vi "PicoCreatePicoMultiBuffers.vi"(1 "Number of Buffers":i32=1, 2 "Buffer and Transfer Settings":T2={"startIndex"=0, "Samples"=1000, "Down Sample Ratio"=1, "Down-Sample Mode"=1} {"Down-Sample Mode" items=["None"=2147483648, "Aggregate"=1, "Decimate"=2, "Average"=4]; "Down Sample Ratio" step=1; "Samples" format="%_6p"}, 3 "enabled array":i16[](array[numeric]), 5 "Data Pointers In":T1, 11 "error in (no error)":errorcluster) -> (6 "Data Pointers":T1, 15 "error out":errorcluster)   [LabVIEW 2024]
doc: "Creates Multiple memory buffers for Pico block and Rapid block examples as configured."
uses:
  PicoBuffers.ctl
panel:
  in  "Dummy enabled array":i16[](array[numeric])=[1, 1, 1, 1, 1, 1, 1, 1, 1, 1]
  # "Samples can be equal to or less\nTotal Pre and Post Trigger Samples"
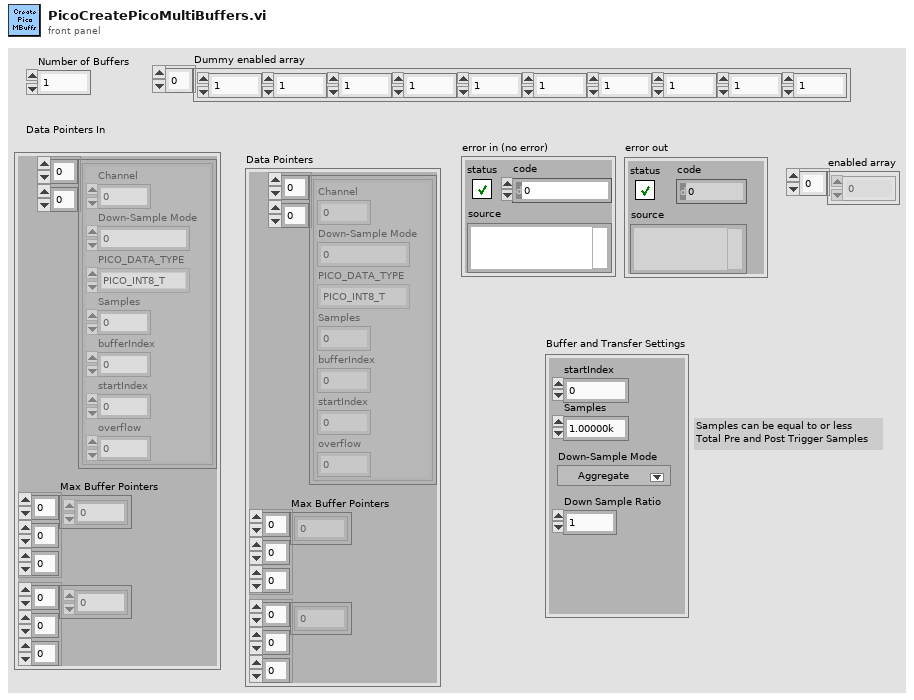
[diagram p1: front panel]
types:
  T1 = typedef "PicoBuffers.ctl" = cluster{"Max Buffer Pointers":u64[][][], "Min Buffer Pointers":u64[][][], "StreamingDataInfo":cluster{"Channel":u32, "Down-Sample Mode":u32, "PICO_DATA_TYPE":enum32{"PICO_INT8_T", "PICO_INT16_T", "PICO_INT32_T", "PICO_UINT32_T", "PICO_INT64_T", ""}, "Samples":i32, "bufferIndex":u64, "startIndex":i32, "overflow":i16}[][]}
  T2 = cluster{"startIndex":u64, "Samples":u64, "Down Sample Ratio":u64, "Down-Sample Mode":u32}
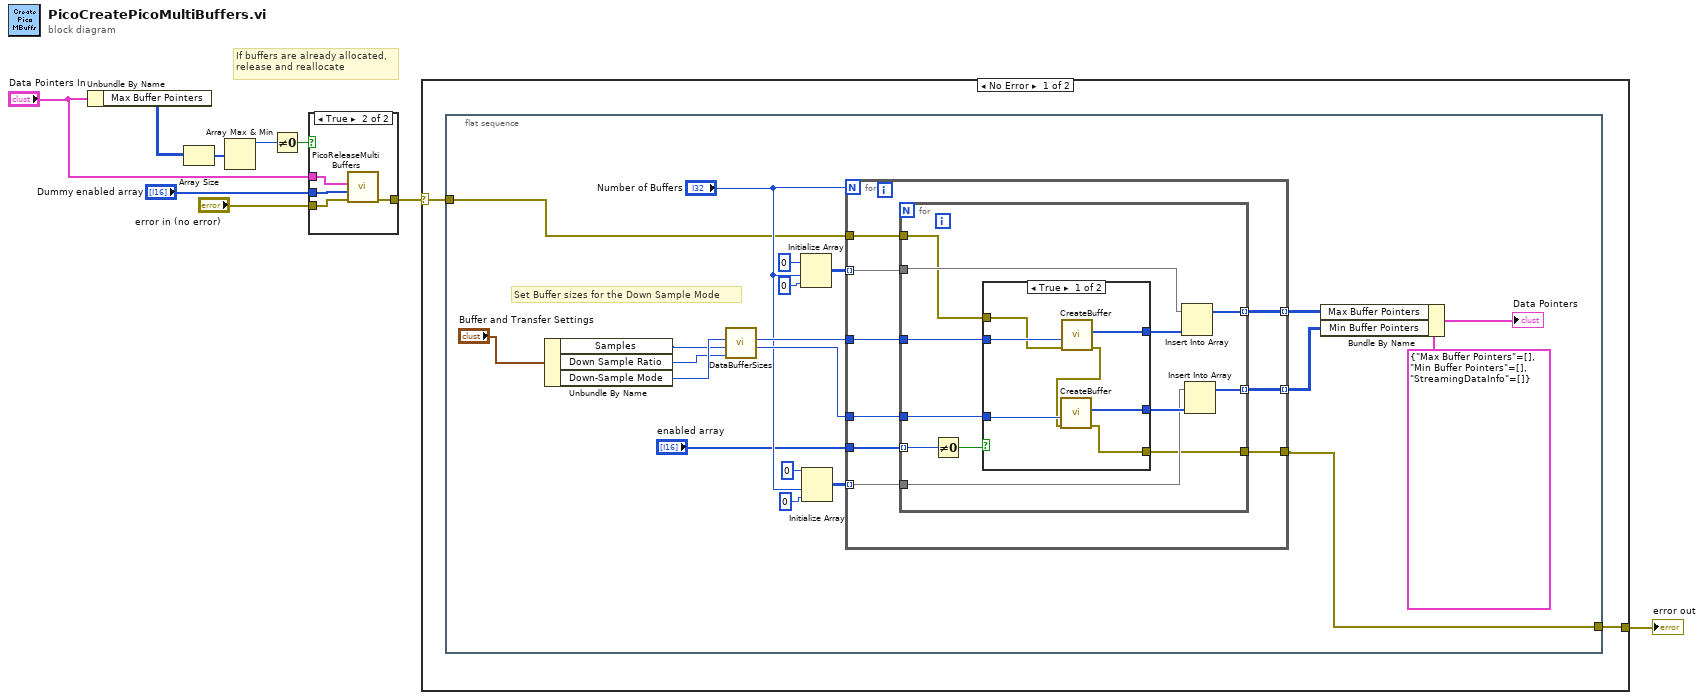
[diagram p0: block diagram]
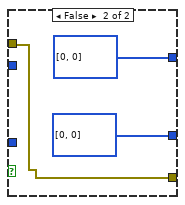
[diagram p3: hidden frame]
diagram:
  # "If buffers are already allocated,\nrelease and reallocate"
  n1 = Unbundle By Name("Data Pointers In") -> ("Max Buffer Pointers"=w6:u64[][][])
  n2 = Array Size(array=w6) -> (size(s)=w8:i32[])
  n3 = Array Max & Min(array=w8) -> (max value=w7:i32)  [unwired: 3 out]
  n4 = Not Equal To 0?(x=w7) -> (x != 0?=w9:bool)
  n5 = case shown="True" w9 {
    tunnel: "error in (no error)" -> [w10 w14]
    tunnel: [w10 w13] -> w2
    tunnel: "Dummy enabled array" -> [_ w12]
    tunnel: "Data Pointers In" -> [_ w11]
    frame False {
    }
    frame True {
      n6 = call "PicoReleaseMultiBuffers.vi"("error in (no error)"=w14, "Enabled array"=w12, "Data Pointers"=w11) -> ("error out"=w13:errorcluster)  [unwired: 7 in, 1 out]
    }
  }
  n7 = case shown="No Error" w2 {
    selector: w2 -> [w16 w68]
    tunnel: [w15 w68] -> w1
    frame No Error {
      n8 = flat-sequence {
        tunnel: w16 -> [w18]
        tunnel: [w17] -> w15
        frame #0 {
          # "Set Buffer sizes for the Down Sample Mode"
          n9 = Unbundle By Name("Buffer and Transfer Settings") -> ("Samples"=w32:u64, "Down Sample Ratio"=w31:u64, "Down-Sample Mode"=w33:u32)
          n10 = call "DataBufferSizes.vi"("Down Sample Ratio"=w31, "Number of Samples"=w32, "Down-Sample Mode"=w33) -> ("min Buffer Size"=w29:i32, "Max Buffer Size"=w30:i32)  [unwired: 7 in]
          n11 = Initialize Array(u64 0 ("element"), "Number of Buffers", 0 ("dimension size")) -> (w34:u64[][])
          n12 = Initialize Array(u64 0 ("element"), "Number of Buffers", 0 ("dimension size")) -> (w26:u64[][])
          n13 = for {
            N: "Number of Buffers" -> [_]
            tunnel: "enabled array" -> [w44]
            tunnel: w30 -> [w45]
            tunnel: w29 -> [w43]
            tunnel: [w42] -> w24 mode=indexing
            tunnel: w34 -> [w41] mode=indexing
            tunnel: w26 -> [w40] mode=indexing
            tunnel: [w39] -> w23 mode=indexing
            tunnel: w18 -> [w38]
            tunnel: [w37] -> w17
            n14 = for {
              tunnel: w45 -> [w57]
              tunnel: w44 -> [w55] mode=indexing
              tunnel: w43 -> [w54]
              tunnel: [w52] -> w42 mode=indexing
              tunnel: w41 -> [w51]
              tunnel: w40 -> [w49]
              tunnel: [w48] -> w39 mode=indexing
              tunnel: w38 -> [w47]
              tunnel: [w46] -> w37
              n15 = Not Equal To 0?(x=w55) -> (x != 0?=w56:bool)
              n16 = case shown="True" w56 {
                tunnel: w57 -> [w63 _]
                tunnel: w54 -> [w64 _]
                tunnel: [w62 u64[] [0, 0]] -> w53
                tunnel: [w61 u64[] [0, 0]] -> w50
                tunnel: w47 -> [w60 w65]
                tunnel: [w58 w65] -> w46
                frame True {
                  n17 = call "CreateBuffer.vi"("error in (no error)"=w60, "Buffer size"=w63) -> ("error out"=w59:errorcluster, "Pointer and BufferSize"=w62:u64[])  [unwired: 8 in]
                  n18 = call "CreateBuffer.vi"("error in (no error)"=w59, "Buffer size"=w64) -> ("error out"=w58:errorcluster, "Pointer and BufferSize"=w61:u64[])  [unwired: 8 in]
                }
                frame False {
                }
              }
              n19 = Insert Into Array(array=w51, new element=w53) -> (w52:u64[])  [unwired: 1 in]
              n20 = Insert Into Array(array=w49, new element=w50) -> (w48:u64[])  [unwired: 1 in]
            }
          }
          n21 = Bundle By Name(cluster=T1 {"Max Buffer Pointers"=[], "Min Buffer Pointers"=[], "StreamingDataInfo"=[]} ("Data Pointers"), "Max Buffer Pointers"=w24, "Min Buffer Pointers"=w23) -> (→"Data Pointers":T1)
        }
      }
    }
    frame Error {
    }
  }
  "error out" <- w1
